vi "controller.vi"(6 "dt (s)":dbl=-1.0 format="%.3f", 7 "PWM Range":cluster{"High PW":dbl, "Low PW":dbl}, 8 "error in (no error)":errorcluster, 9 "FS Data":dbl, 10 "Setpoint":dbl, 11 "PID gains":T1={"proportional gain (Kc)"=1.0, "integral time (Ti, min)"=0.01, "derivative time (Td, min)"=0.0} {"derivative time (Td, min)" format="%.3f"; "integral time (Ti, min)" format="%.3f"; "proportional gain (Kc)" format="%.3f"}) -> (0 "error out":errorcluster, 2 "Uncoerced Output":dbl, 3 "Output":dbl)   [LabVIEW 2020]
uses:
  <vilib>/addons/control/pid/pid.llb/PID (DBL).vi
  <vilib>/addons/control/pid/NI_PID_pid.lvlib
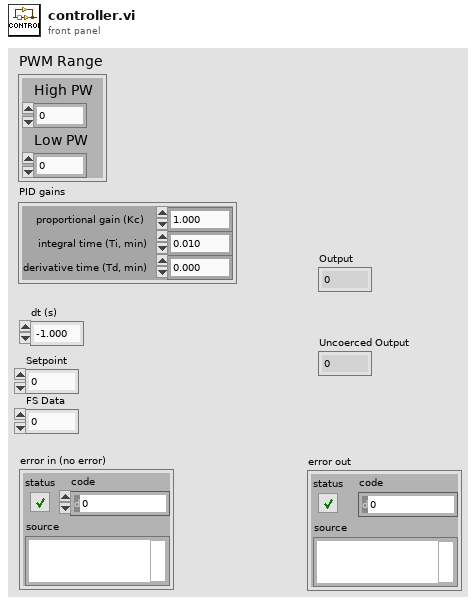
[diagram p1: front panel]
types:
  T1 = cluster{"proportional gain (Kc)":dbl, "integral time (Ti, min)":dbl, "derivative time (Td, min)":dbl}
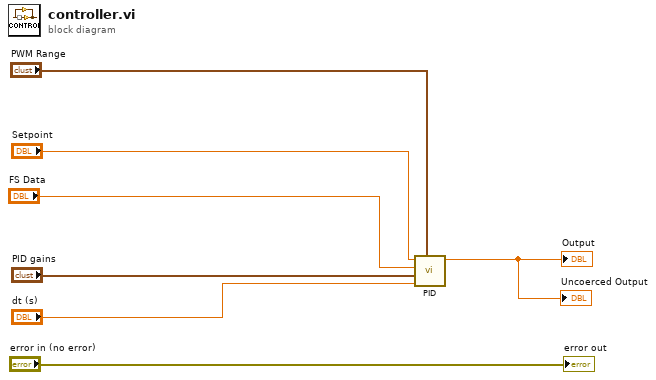
[diagram p0: block diagram]
diagram:
  n1 = call-poly <vilib>:"PID.vi"("output range"="PWM Range", "dt (s)"="dt (s)", "PID gains"="PID gains", "process variable"="FS Data", "setpoint"="Setpoint") -> ("output"=→"Output" →"Uncoerced Output":dbl)  [unwired: 5 in, 1 out]
  "error out" <- "error in (no error)"
